vi "Handle Error.vi"(7 "Stop on Unhandled Error (T)":bool=TRUE, 8 "error in":errorcluster, 11 "SMO.Dictionary":refnum<class "SMO.Dictionary.lvclass">) -> (0 "handling error":errorcluster, 2 "Unhandled error":errorcluster, 3 "SMO.Dictionary out":refnum<class "SMO.Dictionary.lvclass">)   [LabVIEW 2013, in "SMO.Dictionary.lvlib" / "SMO.Dictionary.lvclass"]
doc: "JKI State Machine Objects (SMO) 1.0.0.11\nJKI - JKI\nCopyright (c) 2016, JKIJKI State Machine Objects (SMO) 1.0.1.12\nJKI - JKI\nCopyright (c) 2016, JKI"
uses:
  SMO.Dictionary.lvclass
  <vilib>/JKI/JKI SMO/SMO/SMO.lvclass
panel:
  # "For instructions on how to use the JKI State Machine Objects, examples and video tutorials, visit:\nhttp://jki.net/state-machine-objects/\n\nJKI State Machine Objects™\nhttp://jki.net/state-machine-objects/\nCopyright (C) 2005-2015, JKI <info@jki.net>\nALL RIGHTS RESERVED"
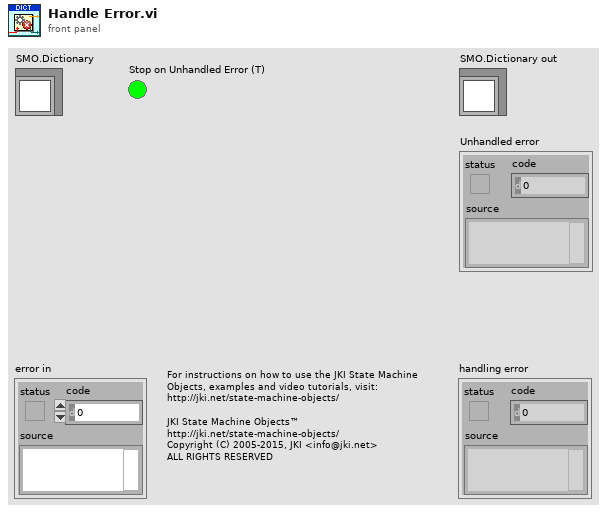
[diagram p1: front panel]
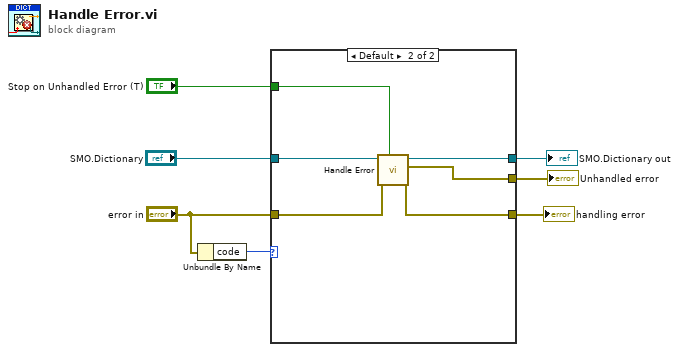
[diagram p0: block diagram]
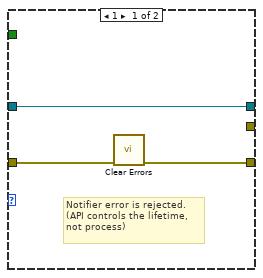
[diagram p2: hidden frame]
diagram:
  n1 = Unbundle By Name("error in") -> ("code"=w1:i32)
  n2 = case shown="Default" w1 {
    tunnel: [_ w16] -> w7
    tunnel: [w10 w15] -> w6
    tunnel: "Stop on Unhandled Error (T)" -> [_ w14]
    tunnel: "SMO.Dictionary" -> [w10 w13]
    tunnel: [w8 w12] -> w3
    tunnel: "error in" -> [w9 w11]
    frame 1 {
      # "Notifier error is rejected.\n(API controls the lifetime, \nnot process)"
      n3 = call <vilib>:"Clear Errors.vi"("error in (no error)"=w9) -> ("error out"=w8:errorcluster)  [unwired: 6 in]
    }
    frame Default {
      n4 = call-parent "Handle Error.vi"("Stop on Unhandled Error (T)"=w14, "error in"=w11, "SMO"=w13) -> ("handling error"=w12:errorcluster, "Unhandled error"=w16:errorcluster, "SMO out"=w15:refnum<class "SMO.Dictionary.lvclass">)  [unwired: 6 in]
    }
  }
  "handling error" <- w3
  "SMO.Dictionary out" <- w6
  "Unhandled error" <- w7
